vi "MongoDB.DocumentSave.vi"(8 "error in (no error)":errorcluster, 11 "MongoDB.Collection in":refnum<class "MongoDB.Collection.lvclass">) -> (0 "error out":errorcluster, 2 "Result":T1, 3 "MongoDB.Collection out":refnum<class "MongoDB.Collection.lvclass">)   [LabVIEW 2014, in "MongoDB.Collection.lvclass"]
uses:
  MongoDB.Collection.lvclass
  C:/Users/Richard/Documents/GitHub/mongo-labview-driver/CSharp/bin/MongoDB.Bson.dll
  CSharp/bin/MongoDB.Bson.dll
  MongoDB.Collection.lvclass/MongoDB.Collection.ctl
  C:/Users/Richard/Documents/GitHub/mongo-labview-driver/CSharp/bin/MongoDB.Driver.Legacy.dll
  CSharp/bin/MongoDB.Driver.Legacy.dll
  C:/Users/Richard/Documents/GitHub/mongo-labview-driver/CSharp/bin/MongoDB.Driver.Core.dll
  CSharp/bin/MongoDB.Driver.Core.dll
panel:
  in  "json":string
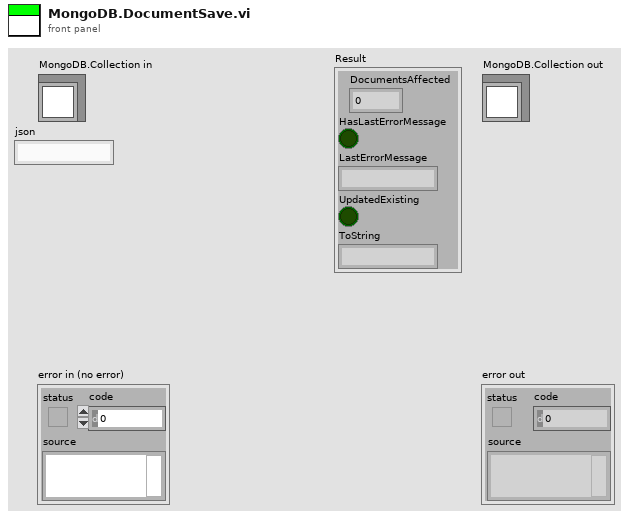
[diagram p1: front panel]
types:
  T1 = cluster{"DocumentsAffected":i64, "HasLastErrorMessage":bool, "LastErrorMessage":string, "UpdatedExisting":bool, "ToString":string}
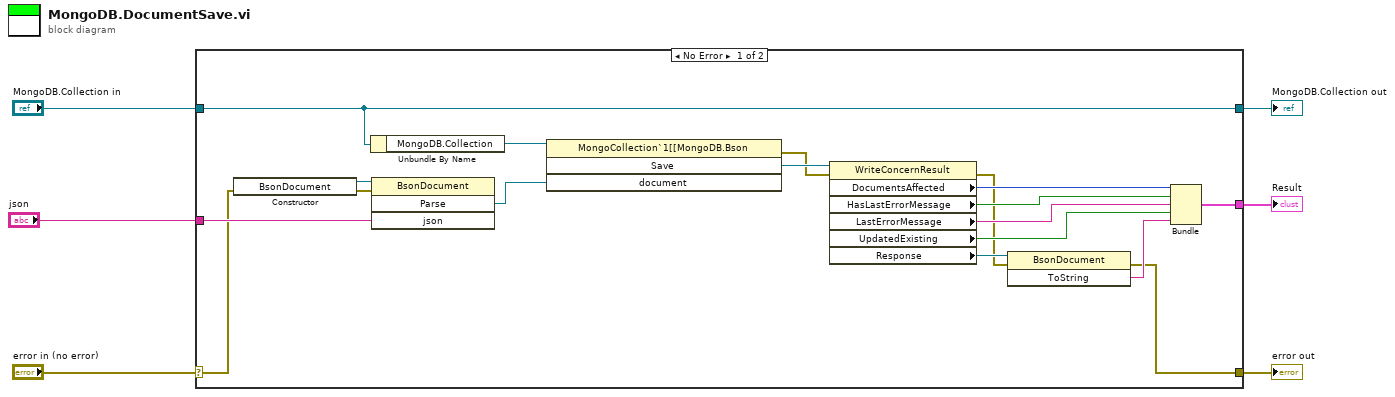
[diagram p0: block diagram]
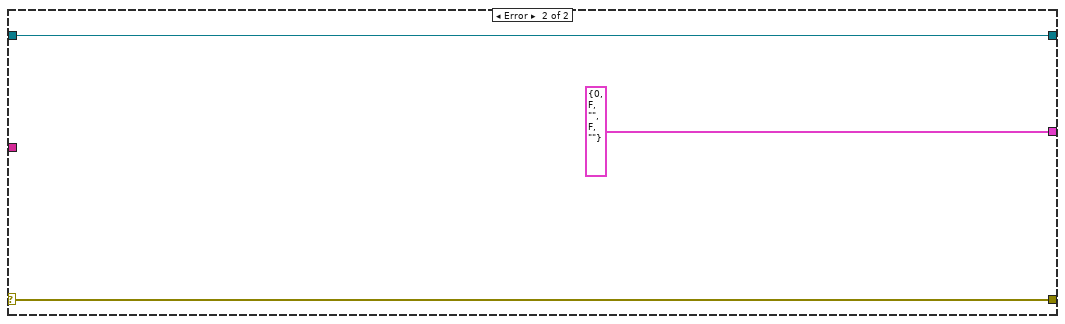
[diagram p2: hidden frame]
diagram:
  n1 = case shown="No Error" "error in (no error)" {
    selector: "error in (no error)" -> [w7 w27]
    tunnel: [w13 w27] -> w5
    tunnel: [w24 w26] -> w3
    tunnel: "MongoDB.Collection in" -> [w24 w26]
    tunnel: [w12 T1 {"DocumentsAffected"=0, "HasLastErrorMessage"=FALSE, "LastErrorMessage"="", "UpdatedExisting"=FALSE, "ToString"=""}] -> w2
    tunnel: "json" -> [w10 _]
    frame No Error {
      n2 = constructor class="BsonDocument"(error in=w7) -> (reference out=w9:refnum<k24>, error out=w8:errorcluster)  [unwired: 2 in, 1 out]
      n3 = Unbundle By Name(w24) -> ("MongoDB.Collection"=w23:refnum<k24>)
      n4 = invoke class="BsonDocument" method="Parse"(reference=w9, error in=w8, "json"=w10) -> ("Parse"=w11:refnum<k24>)  [unwired: 1 in, 3 out]
      n5 = invoke class="MongoCollection`1[[MongoDB.Bson" method="Save"(reference=w23, "document"=w11) -> (error out=w21:errorcluster, "Save"=w22:refnum<k24>)  [unwired: 2 in, 2 out]
      n6 = property class="WriteConcernResult"(reference=w22, error in=w21) -> (error out=w14:errorcluster, "DocumentsAffected"=w20:i64, "HasLastErrorMessage"=w19:bool, "LastErrorMessage"=w18:string, "UpdatedExisting"=w17:bool, "Response"=w16:refnum<k24>)  [unwired: 1 out]
      n7 = invoke class="BsonDocument" method="ToString"(reference=w16, error in=w14) -> (error out=w13:errorcluster, "ToString"=w15:string)  [unwired: 1 in, 1 out]
      n8 = Bundle("DocumentsAffected"=w20, "HasLastErrorMessage"=w19, "LastErrorMessage"=w18, "UpdatedExisting"=w17, "ToString"=w15) -> (w12:T1)  [unwired: 1 in]
    }
    frame Error {
    }
  }
  "error out" <- w5
  "MongoDB.Collection out" <- w3
  "Result" <- w2
